vi "file_import.vi"(8 "error in (no error)":errorcluster, 11 "path in":path) -> (0 "error out":errorcluster, 3 "path out":path)   [LabVIEW 2017, in "rpacini_toml.lvlib"]
uses:
  rpacini_toml.lvlib
  fg_action.ctl
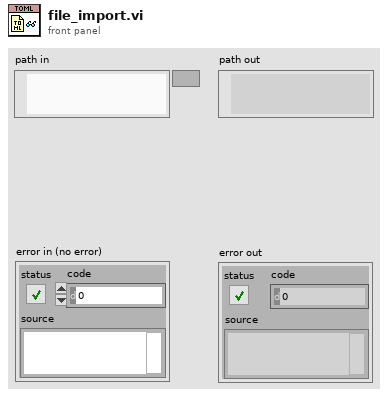
[diagram p1: front panel]
types:
  T1 = typedef "rpacini_toml.lvlib/fg_action.ctl" = enum8{"null", "get", "set", "pop", "import", "export", "drop", "sections", "keys", "remove"}
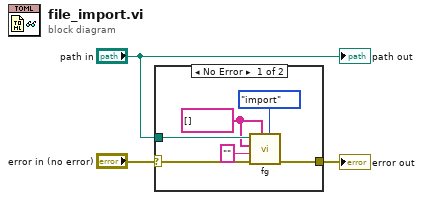
[diagram p0: block diagram]
diagram:
  n1 = case shown="No Error" "error in (no error)" {
    selector: "error in (no error)" -> [w9 w10]
    tunnel: [w8 w10] -> w2
    tunnel: "path in" -> [w7 _]
    frame No Error {
      w4 = string[] [] ("section")
      n2 = call "fg.vi"("action"=fg_action."import", "section"=w4, "error in (no error)"=w9, "value in"="", "key"=w4, "path in"=w7) -> ("error out"=w8:errorcluster)  [unwired: 2 in, 3 out]
    }
    frame Error {
    }
  }
  "error out" <- w2
  "path out" <- "path in"
